vi "Sub Initialize.vi"(8 "error in (no error)":errorcluster, 11 "Spectrum Recorder in":refnum<class "Spectrum Recorder too.lvclass">) -> (0 "error out":errorcluster, 2 "Initialize Result":refnum<class "Acquired Result.lvclass">, 3 "Spectrum Recorder out":refnum<class "Spectrum Recorder too.lvclass">)   [LabVIEW 2016, in "Spectrum Recorder too.lvclass"]
uses:
  Spectrum Recorder too.lvclass
  C:/github/LabActor/Worker/Worker.lvclass
  C:/github/LabActor/Instrument Actor/Instrument Actor.lvclass
  NHMFL_Core/Libraries/Instruments/Results/Acquired Result/Acquired Result.lvclass
  Worker/Worker.lvclass/Worker.ctl
  Spectrum Recorder too.lvclass/Spectrum Recorder too.ctl
  NHMFL_Core/Libraries/Instruments/Instrument Driver/Worker State.ctl
  Template Module/Write State.vi
  Template Module/Read State.vi
  Read Spectrum Recorder Configuration.vi
  Instrument Actor/Instrument Actor.lvclass
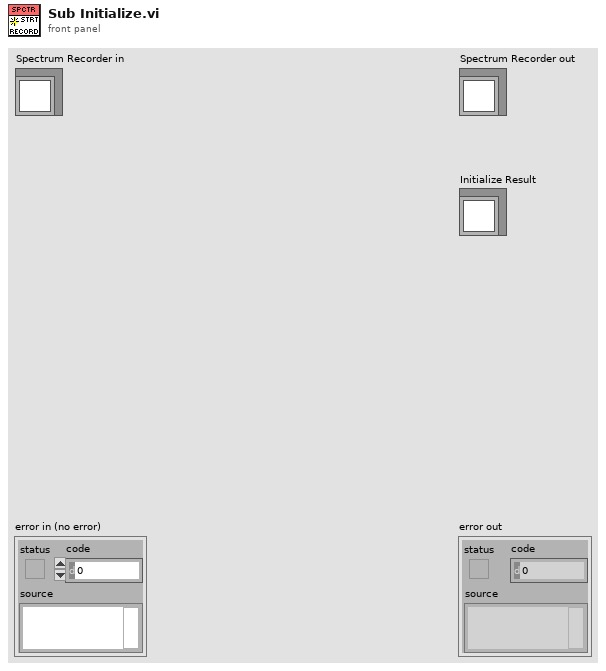
[diagram p1: front panel]
types:
  T1 = typedef "Worker State.ctl" = enum16{"Idle", "Starting", "Working", "Stopping"}
  T2 = typedef "Spectrum Configuration.ctl" = cluster{"Start frequency":dbl, "End frequency":dbl, "Coarse step":dbl, "Step duration":dbl, "Red Pitaya address":string, "Open plot \non start":bool, "Fine region centers":dbl[], "Regions width":dbl, "Fine step":dbl, "Pause between scans":dbl, "Clear rgs on start":bool}
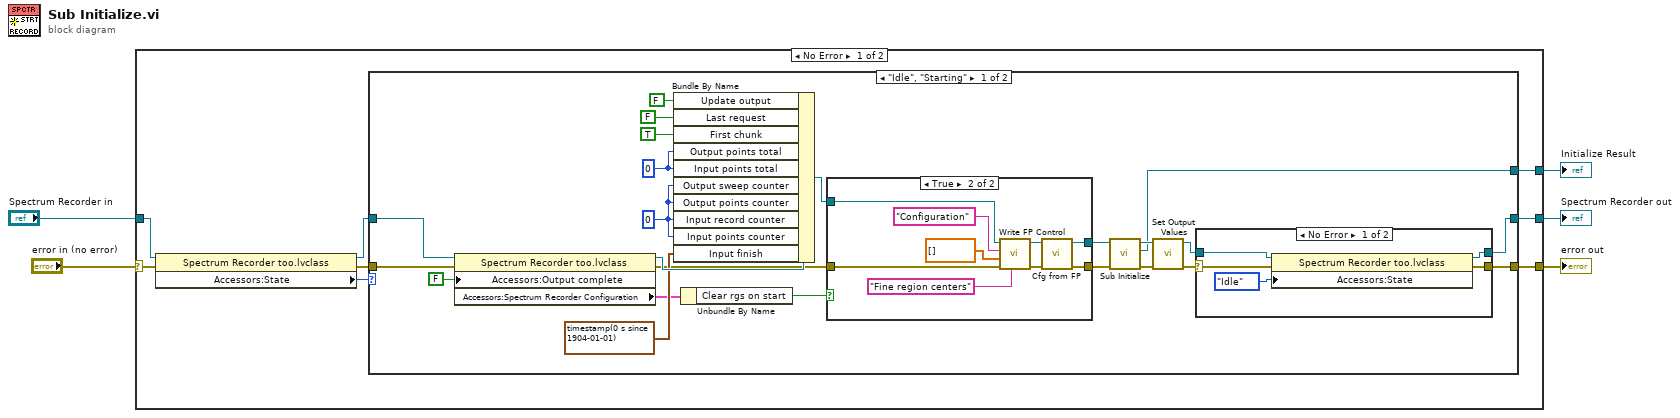
[diagram p0: block diagram]
diagram:
  n1 = case shown="No Error" "error in (no error)" {
    selector: "error in (no error)" -> [w8 w58]
    tunnel: [w11 w58] -> w4
    tunnel: [w13 w57] -> w2
    tunnel: "Spectrum Recorder in" -> [w12 w57]
    tunnel: [w6 _] -> w1
    frame No Error {
      n2 = property class="Spectrum Recorder too.lvclass"(reference=w12, error in=w8) -> (reference out=w10:refnum<class "Spectrum Recorder too.lvclass">, error out=w7:errorcluster, "Accessors:State"=w9:T1)
      n3 = case shown="\"Idle\", \"Starting\"" w9 {
        tunnel: w10 -> [w29 w56]
        tunnel: [w31 w56] -> w13
        tunnel: w7 -> [w27 w55]
        tunnel: [w36 w55] -> w11
        tunnel: [w23 _] -> w6
        frame "Idle", "Starting" {
          w30 = i64 0 ("Output points total")
          w35 = 0 ("Output sweep counter")
          n4 = property class="Spectrum Recorder too.lvclass"(reference=w29, error in=w27, "Accessors:Output complete"=FALSE ("Output complete")) -> (reference out=w28:refnum<class "Spectrum Recorder too.lvclass">, error out=w17:errorcluster, "Accessors:Spectrum Recorder Configuration"=w20:T2)
          n5 = Bundle By Name(cluster=w28, "Update output"=FALSE, "Last request"=FALSE, "First chunk"=TRUE, "Output points total"=w30, "Input points total"=w30, "Output sweep counter"=w35, "Output points counter"=w35, "Input record counter"=w35, "Input points counter"=w35, "Input finish"=timestamp(0 s since 1904-01-01)) -> (w18:refnum<class "Spectrum Recorder too.lvclass">)
          n6 = Unbundle By Name(w20) -> ("Clear rgs on start"=w19:bool)
          n7 = case shown="True" w19 {
            tunnel: w18 -> [w38 w47]
            tunnel: w17 -> [w37 w44]
            tunnel: [w37 w39] -> w16
            tunnel: [w38 w40] -> w15
            frame False {
            }
            frame True {
              n8 = call-dynamic "Write FP Control.vi"("Field name"="Fine region centers", "error in (no error)"=w44, "Control Value"=dbl[] [], "Control Name"="Configuration", "Measure Object in"=w47) -> ("error out"=w41:errorcluster, "Measure Object out"=w42:refnum<class "Spectrum Recorder too.lvclass">)  [unwired: 5 in]
              n9 = call-dynamic "Cfg from FP.vi"("error in (no error)"=w41, "Measure Object in"=w42) -> ("error out"=w39:errorcluster, "Measure Object out"=w40:refnum<class "Spectrum Recorder too.lvclass">)  [unwired: 8 in]
            }
          }
          n10 = call-parent "Sub Initialize.vi"("error in (no error)"=w16, "Instrument Recorder in"=w15) -> ("error out"=w24:errorcluster, "Initialize Result"=w23:refnum<class "Acquired Result.lvclass">, "Instrument Recorder out"=w25:refnum<class "Spectrum Recorder too.lvclass">)  [unwired: 7 in]
          n11 = call-dynamic "Set Output Values.vi"("error in (no error)"=w24, "Spectrum Recorder in"=w25) -> ("error out"=w33:errorcluster, "Spectrum Recorder out"=w32:refnum<class "Spectrum Recorder too.lvclass">)  [unwired: 8 in]
          n12 = case shown="No Error" w33 {
            selector: w33 -> [w52 w53]
            tunnel: [w49 w53] -> w36
            tunnel: w32 -> [w51 w54]
            tunnel: [w50 w54] -> w31
            frame No Error {
              n13 = property class="Spectrum Recorder too.lvclass"(reference=w51, error in=w52, "Accessors:State"=Worker_State."Idle" ("State")) -> (reference out=w50:refnum<class "Spectrum Recorder too.lvclass">, error out=w49:errorcluster)
            }
            frame Error {
            }
          }
        }
        frame "Working", Default {
        }
      }
    }
    frame Error {
    }
  }
  "error out" <- w4
  "Spectrum Recorder out" <- w2
  "Initialize Result" <- w1
